vi "ContextHelp_CheckHelpForControl.vi"(0 "Ctl Refnum":refnum<vi>, 1 "Help":bool, 5 "error in (no error)":errorcluster) -> (19 "error out":errorcluster)   [LabVIEW 2016]
uses:
  <resource>/Framework/Providers/Open_GDS/UML/ContextHelp/ContextHelp_HelpTexts.ctl
panel:
  in  "HelpText":T1
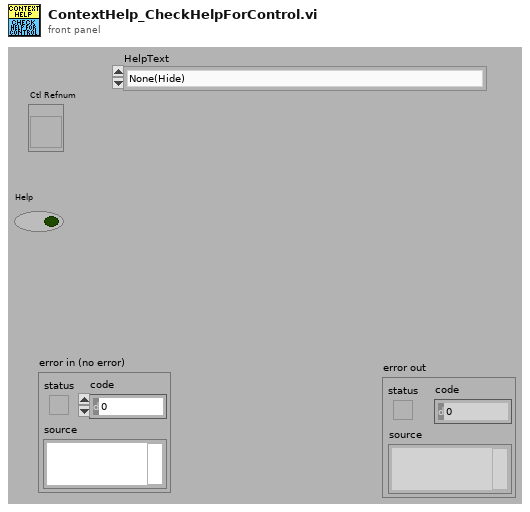
[diagram p1: front panel]
types:
  T1 = typedef "ContextHelp_HelpTexts.ctl" = enum16{"None(Hide)", "Default", "Help", "Welcome", "GettingStarted", "ClassDiagram_Help", "SequenceDiagram_Help", "UseCaseDiagram_Help", "BSelect", "BClass", "BInterface", "BPackage", "BNote", "BDependency", "BInheritance", "BInterfaceImplementation", "BAssociation", "BAggregation", "BCompAggregation", "BNoteConnector", "BObject", "BActionBar", "BCall", "BSystem", "BActor", "BUseCase", "BGeneralization", "BIncludes", "BExtends", "BUseCaseDiagramAssociation", "ClassRelationshipEdge editDialog_Bent Style", "ClassRelationshipEdge editDialog_RelationType", "ClassRelationshipEdge editDialog_Reverse association", "ClassRelationshipEdge editDialog_Start label", "ClassRelationshipEdge editDialog_Middle label", "ClassRelationshipEdge editDialog_End label", "UMLEditor reversedEngineering_Pathes", "ReversedEngineering StateReverseDialog_Help", "ReversedEngineering StateQueuedSettings_Help", "UMLEditor reversedEngineering_AddTopVIs", "UMLEditor reversedEngineering_AddClasses", "UMLEditor reversedEngineering_AddDirs", "UMLEditor reversedEngineering_Recursively", "UMLEditor reversedEngineering_Remove", "UMLEditor reversedEngineering_ClearList", "UMLEditor reversedEngineering_HideSubAss", "UMLEditor reversedEngineering_CreateTypes", "UMLEditor reversedEngineering_OnlyInheritance", "UMLEditor reversedEngineering_CreateApplication", "UMLEditor reversedEngineering_OK", "UMLEditor reversedEngineering_Cancel", "UMLEditor reversedEngineering_Help", "UMLEditor createWizardScriptFile_ScriptfilePath", "UMLEditor createWizardScriptFile_ClassPath", "UMLEditor createWizardScriptFile_Use", "UMLEditor createWizardScriptFile_PrivateDirName", "UMLEditor createWizardScriptFile_DirAppend", "UMLEditor createWizardScriptFile_Separator Character", "UMLEditor createWizardScriptFile_OK", "UMLEditor createWizardScriptFile_Cancel", "UMLEditor createWizardScriptFile_Help", "ClassNode editDialog_Class Name", "InterfaceNode editDialog_Class Name", "ClassNode editDialog_Attribute", "ClassNode editDialog_Methods", "InterfaceNode editDialog_Methods", "ClassNode editDialog_connection", "InterfaceNode editDialog_connection", "ClassNode editDialog_StereoType", "ClassNode editDialog_ShowAttrib", "ClassNode editDialog_ShowMethods", "ClassNode editDialog_ClassPath", "ClassNode editDialog_AddAttribute", "ClassNode editDialog_AddMethod", "InterfaceNode editDialog_AddMethod", "ClassNode AttributeGuide_AttributeName", "ClassNode AttributeGuide_Array?", "ClassNode AttributeGuide_Data Type", "ClassNode AttributeGuide_RefName", "ClassNode AttributeGuide_Preview", "ClassNode AttributeGuide_OK", "ClassNode AttributeGuide_Cancel", "ClassNode MethodGuide_Visibility", "ClassNode MethodGuide_Method Name", "ClassNode MethodGuide_Preview", "ClassNode MethodGuide_OK", "ClassNode MethodGuide_Cancel", "CallNode EditCallProperties_AllButtons", "ObjectNode EditObjectlProperties_AllButtons", "ActorNode EditActorProperties_AllButtons", "UseCaseRelationshipNode EditUseCaselProperties_AllButtons", "UseCaseNode EditUseCaselProperties_AllButtons", "SystemNode EditSystemProperties_AllButtons", "ReversedEngineering UpdateAttributes_AllButtons", "StateNode editDialog_AllButtons", "StateTransition editDialog_AllButtons", "ArrangeNodes Main_Picture", "ArrangeNodes Main_Zoom", "ArrangeNodes Main_Auto Zoom", "ArrangeNodes Main_shorten", "ArrangeNodes Main_Min Length", "ArrangeNodes Main_Max Length", "ArrangeNodes Main_increase", "ArrangeNodes Main_decrease", "ArrangeNodes Main_Shake", "ArrangeNodes Main", "BState", "BInitialState", "BFinalState", "BStateTransition", "StateDiagram_Help", "StateDiagram_PropertiesAllButtons", "ReversedEngineering StateReverseDialog_ClearStates", "ReversedEngineering StateReverseDialog_UseQueuedStateMachines", "ReversedEngineering StateReverseDialog_QueuedSettings", "ReversedEngineering StateReverseDialog_SearchForVIs", "ReversedEngineering StateReverseDialog_SearchCriteria", "OptionsDialog_ClassBasePath", "OptionsDialog_VIPath", "OptionsDialog_ApplicationPath", "OptionsDialog_WizDir", "OptionsDialog_IniFilePath", "OptionsDialog_DefineColors", "OptionsDialog_Help", "OptionsDialog_CreateTypes", "ClassRelationshipEdge editDialog_SplitWire"}
  T2 = typedef "ContextHelp_ShowType.ctl" = cluster{"Header":string, "Picture":picture, "Text":string}
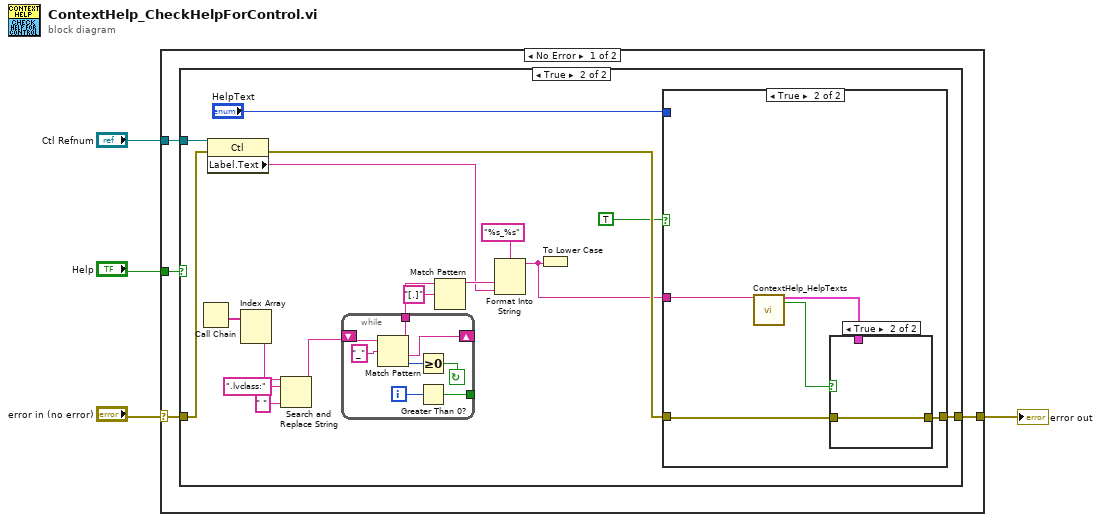
[diagram p0: block diagram]
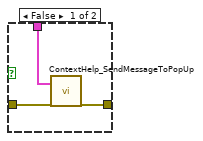
[diagram p4: hidden frame]
diagram:
  n1 = case shown="No Error" "error in (no error)" {
    selector: "error in (no error)" -> [w7 w45]
    tunnel: [w6 w45] -> w3
    tunnel: "Help" -> [w8 _]
    tunnel: "Ctl Refnum" -> [w5 _]
    frame No Error {
      n2 = case shown="True" w8 {
        tunnel: w7 -> [w9 w24]
        tunnel: [w9 w18] -> w6
        tunnel: w5 -> [_ w26]
        frame False {
        }
        frame True {
          n3 = Call Chain() -> (call chain=w25:string[])
          n4 = property class="Ctl"(reference=w26, error in=w24) -> (error out=w17:errorcluster, "Label.Text"=w19:string)  [unwired: 1 out]
          n5 = Index Array(array=w25) -> (element #2=w11:string)  [unwired: 2 in, 1 out]
          n6 = Search and Replace String(input string=w11, search string=".lvclass:", replace string=" " ("replace string (\"\")")) -> (result string=w10:string)  [unwired: 5 in, 3 out]
          n7 = while {
            shift-right: [w41] -> _
            shift-left: w10 -> [w40]
            tunnel: [w38] -> _
            tunnel: [w37] -> w23
            i -> [w39]
            stop <- w42 continue-if-true
            n8 = Match Pattern(string=w40, regular expression="_") -> (before substring=w37:string, after substring=w41:string, offset past match=w43:i32)  [unwired: 2 out]
            n9 = Greater Or Equal To 0?(x=w43) -> (x >= 0?=w42:bool)
            n10 = Greater Than 0?(x=w39) -> (x > 0?=w38:bool)
          }
          n11 = Match Pattern(string=w23, regular expression="[.]") -> (before substring=w20:string)  [unwired: 4 out]
          n12 = Format Into String(format string="%s_%s", w20, w19) -> (resulting string=w15:string)  [unwired: 2 in, 1 out]
          n13 = To Lower Case(string=w15) -> ()  [unwired: 1 out]
          n14 = case shown="True" TRUE {
            tunnel: [w27 w30] -> w18
            tunnel: w17 -> [w27 w31]
            tunnel: "HelpText" -> [_ _]
            tunnel: w15 -> [_ w29]
            frame False {
              # "This control has no Help Text"
            }
            frame True {
              n15 = call <resource>:"ContextHelp_HelpTexts.vi"("HelpText (enum or string)"=w29) -> ("HelpOut"=w32:T2, "NotFound"=w28:bool)  [unwired: 17 out]
              n16 = case shown="True" w28 {
                tunnel: w32 -> [w35 _]
                tunnel: w31 -> [w34 w36]
                tunnel: [w33 w36] -> w30
                frame False {
                  n17 = call <resource>:"ContextHelp_SendMessageToPopUp.vi"("PopUpMessage"=w35, "error in (no error)"=w34) -> ("error out"=w33:errorcluster)  [unwired: 17 out]
                }
                frame True {
                }
              }
            }
          }
        }
      }
    }
    frame Error {
    }
  }
  "error out" <- w3
